vi "EVENTS(SubVI).vi"(1 "concatenated string":string) -> (0 "Events":string)   [LabVIEW 2014]
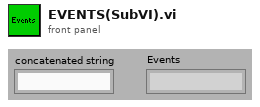
[diagram p1: front panel]
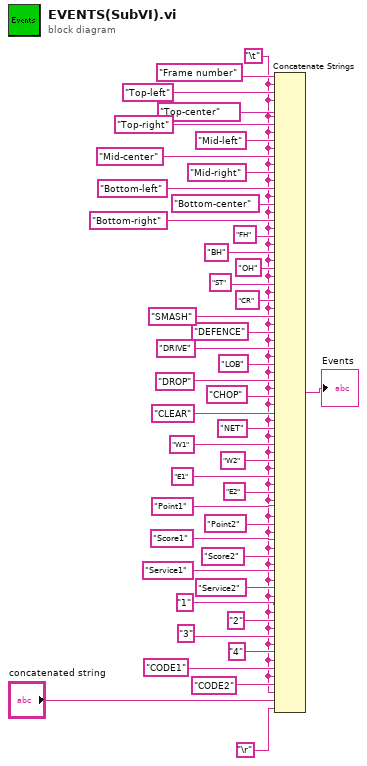
[diagram p0: block diagram]
diagram:
  w3 = "\t"
  n1 = Concatenate Strings("Frame number" ("string"), w3, "Top-left" ("string"), w3, "Top-center" ("string"), w3, "Top-right" ("string"), w3, "Mid-left" ("string"), w3, "Mid-center" ("string"), w3, "Mid-right" ("string"), w3, "Bottom-left" ("string"), w3, "Bottom-center" ("string"), w3, "Bottom-right" ("string"), w3, "FH" ("string"), w3, "BH" ("string"), w3, "OH" ("string"), w3, "ST" ("string"), w3, "CR" ("string"), w3, "SMASH" ("string"), w3, "DEFENCE" ("string"), w3, "DRIVE" ("string"), w3, "LOB" ("string"), w3, "DROP" ("string"), w3, "CHOP" ("string"), w3, "CLEAR" ("string"), w3, "NET" ("string"), w3, "W1" ("string"), w3, "W2" ("string"), w3, "E1" ("string"), w3, "E2" ("string"), w3, "Point1" ("string"), w3, "Point2" ("string"), w3, "Score1" ("string"), w3, "Score2" ("string"), w3, "Service1" ("string"), w3, "Service2" ("string"), w3, "1" ("string"), w3, "2" ("string"), w3, "3" ("string"), w3, "4" ("string"), w3, "CODE1" ("string"), w3, "CODE2" ("string"), w3, "concatenated string", "\r") -> (→"Events":string)
